vi "电压输出采集.vi"() -> ()   [LabVIEW 2014]
uses:
  <vilib>/DAQmx/create/channels.llb/DAQmx Create Channel (AO-Voltage-Basic).vi
  <vilib>/DAQmx/write.llb/DAQmx Write (Analog DBL 1Chan 1Samp).vi
  <vilib>/DAQmx/create/channels.llb/DAQmx Create Channel (AI-Voltage-Basic).vi
  <vilib>/DAQmx/read.llb/DAQmx Read (Analog DBL 1Chan 1Samp).vi
panel:
  in  "输入通道":tag
  out "测量电压":dbl caption="数据" format="%0.2f"
  in  "停止测量":bool
  in  "停止输出":bool
  in  "输出电压":dbl format="%0.2f"
  in  "输出通道":tag
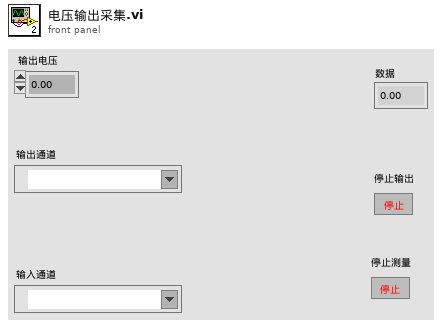
[diagram p1: front panel]
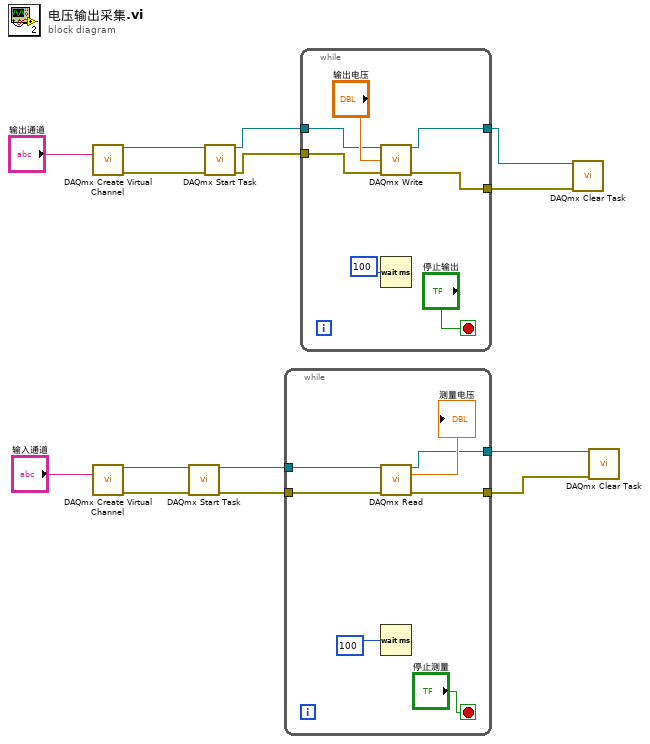
[diagram p0: block diagram]
diagram:
  n1 = call-poly <vilib>:"DAQmx Create Virtual Channel.vi"("physical channels"="输出通道") -> ("task out"=w13:refnum<k21>, "error out"=w12:errorcluster)  [unwired: 13 in]
  n2 = call-poly <vilib>:"DAQmx Create Virtual Channel.vi"("physical channels"="输入通道") -> ("task out"=w7:refnum<k21>, "error out"=w6:errorcluster)  [unwired: 13 in]
  n3 = call <vilib>:"DAQmx Start Task.vi"("task/channels in"=w7, "error in"=w6) -> ("task out"=w5:refnum<k21>, "error out"=w4:errorcluster)  [unwired: 12 in]
  n4 = call <vilib>:"DAQmx Start Task.vi"("task/channels in"=w13, "error in"=w12) -> ("task out"=w11:refnum<k21>, "error out"=w10:errorcluster)  [unwired: 12 in]
  n5 = while {
    tunnel: w5 -> [w18]
    tunnel: w4 -> [w17]
    tunnel: [w16] -> w3
    tunnel: [w15] -> w2
    stop <- "停止测量" stop-if-true
    n6 = call-poly <vilib>:"DAQmx Read.vi"("task/channels in"=w18, "error in"=w17) -> ("task out"=w16:refnum<k21>, "data"=→"测量电压":dbl, "error out"=w15:errorcluster)  [unwired: 11 in]
    n7 = Wait (ms)(milliseconds to wait=100) -> ()  [unwired: 1 out]
  }
  n8 = while {
    tunnel: w11 -> [w25]
    tunnel: w10 -> [w24]
    tunnel: [w23] -> w9
    tunnel: [w22] -> w8
    stop <- "停止输出" stop-if-true
    n9 = call-poly <vilib>:"DAQmx Write.vi"("task/channels in"=w25, "data"="输出电压", "error in"=w24) -> ("task out"=w23:refnum<k21>, "error out"=w22:errorcluster)  [unwired: 10 in, 1 out]
    n10 = Wait (ms)(milliseconds to wait=100) -> ()  [unwired: 1 out]
  }
  n11 = call <vilib>:"DAQmx Clear Task.vi"("task in"=w9, "error in"=w8) -> ()  [unwired: 13 in, 1 out]
  n12 = call <vilib>:"DAQmx Clear Task.vi"("task in"=w3, "error in"=w2) -> ()  [unwired: 13 in, 1 out]
